vi "GetClassHierarchy.vi"(8 "error in (no error)":errorcluster, 11 "object":refnum<class>) -> (0 "error out":errorcluster, 3 "ClassHierarchy":refnum<class>[](array[class]))   [LabVIEW 2020, in "ORM.lvlib" / "TypeMap.lvclass"]
uses:
  TypeMap.lvclass
  TypeMap.lvclass/TypeMap.ctl
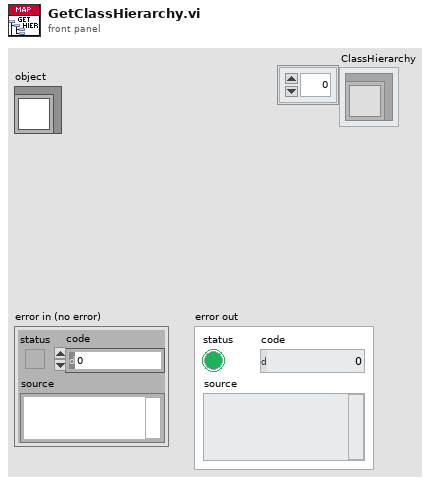
[diagram p1: front panel]
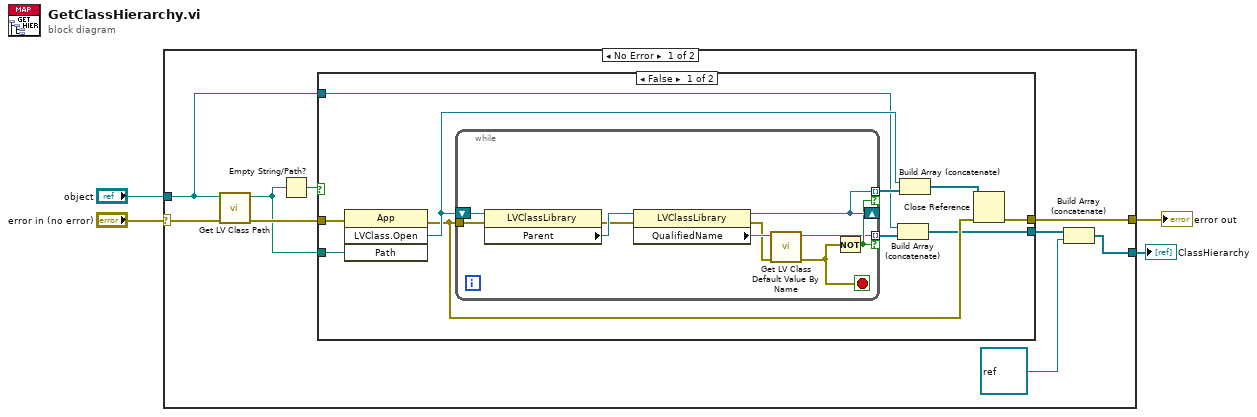
[diagram p0: block diagram]
diagram:
  n1 = case shown="No Error" "error in (no error)" {
    selector: "error in (no error)" -> [w11 w35]
    tunnel: [w10 w35] -> w3
    tunnel: [w7 _] -> w1
    tunnel: "object" -> [w6 _]
    frame No Error {
      n2 = call <vilib>:"Get LV Class Path.vi"("error in (no error)"=w11, "object"=w6) -> ("error out"=w13:errorcluster, "class path"=w9:path)  [unwired: 8 in]
      n3 = Empty String/Path?(string/path=w9) -> (empty?=w8:bool)
      n4 = case shown="False" w8 {
        tunnel: w13 -> [w23 w34]
        tunnel: [w15 _] -> w12
        tunnel: [w17 w34] -> w10
        tunnel: w9 -> [w16 _]
        tunnel: w6 -> [w14 _]
        frame False {
          n5 = invoke class="App" method="LVClass.Open"(error in=w23, "Path"=w16) -> (error out=w18:errorcluster, "LVClass.Open"=w20:refnum<vi>)  [unwired: 2 in, 2 out]
          n6 = while {
            tunnel: w18 -> [w32]
            tunnel: [w26] -> w22 mode=indexing if=w28
            shift-right: [w29] -> _
            shift-left: w20 -> [w33]
            tunnel: [w29] -> w21 mode=indexing if=w28
            stop <- w24 stop-if-true
            n7 = property class="LVClassLibrary"(reference=w33, error in=w32) -> (error out=w30:errorcluster, "Parent"=w31:refnum<vi>)  [unwired: 1 out]
            n8 = property class="LVClassLibrary"(reference=w31, error in=w30) -> (reference out=w29:refnum<vi>, error out=w25:errorcluster, "QualifiedName"=w27:string)
            n9 = call <vilib>:"Get LV Class Default Value By Name.vi"("error in (no error)"=w25, "class name"=w27) -> ("error out"=w24:errorcluster, "object"=w26:refnum<class>)  [unwired: 8 in]
            n10 = Not(x=w24) -> (.not. x?=w28:bool)
          }
          n11 = Build Array (concatenate)(w14, w22) -> (w15:refnum<class>[])
          n12 = Build Array (concatenate)(w20, w21) -> (w19:refnum<vi>[])
          n13 = Close Reference(reference=w19, error in (no error)=w18) -> (error out=w17:errorcluster)
        }
        frame True {
        }
      }
      n14 = Build Array (concatenate)(w12, refnum<class> refnum ("object")) -> (w7:refnum<class>[])
    }
    frame Error {
    }
  }
  "error out" <- w3
  "ClassHierarchy" <- w1
